vi "(SubVI) Notch Filter.vi"(1 "Notch Filter On?":bool, 2 "Data":dbl[](array[numeric]), 3 "Notch freq. (Hz)":dbl, 5 "Sampling rate (Hz)":i32) -> (7 "Filtered Data":dbl[](array[numeric]))   [LabVIEW 2014]
uses:
  <vilib>/Analysis/3filter.llb/Filter Passband Type.ctl
  <vilib>/Analysis/3filter.llb/Bessel Filter (DBL).vi
  <vilib>/Analysis/NI_AALBase.lvlib
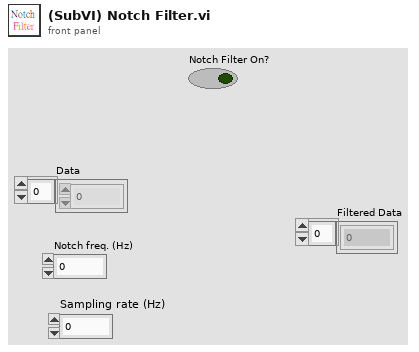
[diagram p1: front panel]
types:
  T1 = typedef "NI_AALBase.lvlib/Filter Passband Type.ctl" = enum32{"Lowpass", "Highpass", "Bandpass", "Bandstop"}
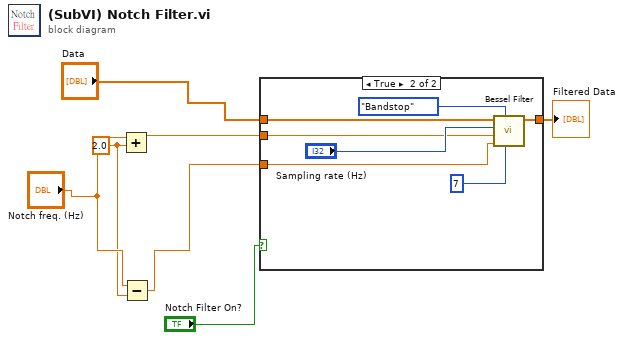
[diagram p0: block diagram]
diagram:
  w3 = 2.0 ("y")
  n1 = Add(x="Notch freq. (Hz)", y=w3) -> (x+y=w2:dbl)
  n2 = Subtract(x="Notch freq. (Hz)", y=w3) -> (x-y=w1:dbl)
  n3 = case shown="True" "Notch Filter On?" {
    tunnel: "Data" -> [w8 w13]
    tunnel: [w8 w12] -> w5
    tunnel: w2 -> [_ w10]
    tunnel: w1 -> [_ w9]
    frame False {
    }
    frame True {
      n4 = call-poly <vilib>:"Bessel Filter.vi"("order"=7, "filter type"=Filter_Passband_Type."Bandstop", "low cutoff freq: fl"=w9, "high cutoff freq: fh"=w10, "sampling freq: fs"="Sampling rate (Hz)", "X"=w13) -> ("Filtered X"=w12:dbl[])  [unwired: 2 in, 1 out]
    }
  }
  "Filtered Data" <- w5
